vi "Text file pattern.vi"(8 "error in":errorcluster, 11 "T in":dbl) -> (0 "error out":errorcluster, 1 "selected path":path, 2 "refnum out":refnum<file>, 3 "T out":dbl)   [LabVIEW 2013]
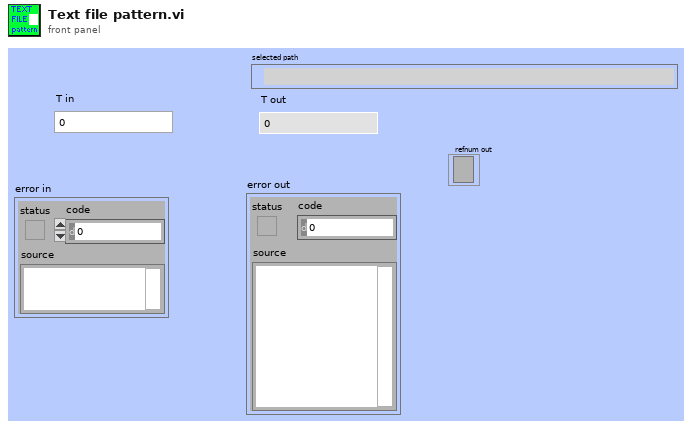
[diagram p1: front panel]
types:
  T1 = enum16{"open", "replace", "create", "open or create", "replace or create", "replace or create with confirmation"}
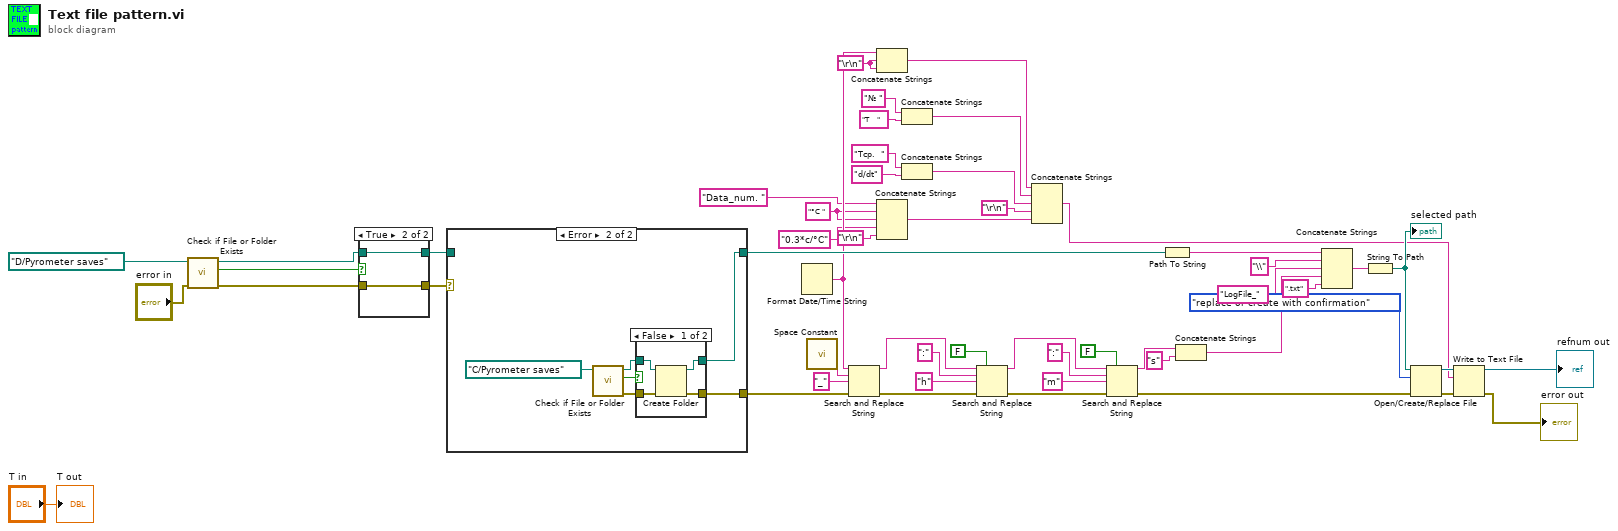
[diagram p0: block diagram]
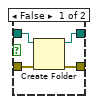
[diagram p4: hidden frame]
diagram:
  w3 = "°C " ("string")
  w8 = "\r\n"
  n1 = call <vilib>:"Check if File or Folder Exists.vi"("error in (no error)"="error in", "path"=path "D:/Pyrometer saves" ("path (use dialog)")) -> ("error out"=w31:errorcluster, "file or folder exists?"=w26:bool, "dup path"=w32:path)  [unwired: 7 out]
  n2 = case shown="True" w26 {
    tunnel: [w57 w59] -> w24
    tunnel: w32 -> [w56 w59]
    tunnel: w31 -> [w55 w58]
    tunnel: [w54 w58] -> w25
    frame False {
      n3 = Create Folder(path (use dialog)=w56, error in=w55) -> (created path=w57:path, error out=w54:errorcluster)  [unwired: 2 out]
    }
    frame True {
    }
  }
  n4 = case shown="Error" w25 {
    tunnel: w24 -> [w60 _]
    tunnel: [w60 w62] -> w23
    tunnel: [_ w61] -> w22
    frame No Error {
    }
    frame Error {
      n5 = call <vilib>:"Check if File or Folder Exists.vi"("path"=path "C:/Pyrometer saves" ("path (use dialog)")) -> ("error out"=w64:errorcluster, "file or folder exists?"=w63:bool, "dup path"=w65:path)  [unwired: 1 in, 7 out]
      n6 = case shown="False" w63 {
        tunnel: [w70 w72] -> w62
        tunnel: w65 -> [w69 w72]
        tunnel: w64 -> [w68 w71]
        tunnel: [w67 w71] -> w61
        frame False {
          n7 = Create Folder(path (use dialog)=w69, error in=w68) -> (created path=w70:path, error out=w67:errorcluster)  [unwired: 2 out]
        }
        frame True {
        }
      }
    }
  }
  n8 = Format Date/Time String() -> (date/time string=w7:string)  [unwired: 3 out]
  n9 = call <vilib>:"Space Constant.vi"() -> ("String"=w46:string)
  n10 = Search and Replace String(input string=w7, search string=w46, replace string="_" ("replace string (\"\")"), error in=w22) -> (result string=w44:string, error out=w30:errorcluster)  [unwired: 6 out]
  n11 = Concatenate Strings(w7, w8, w8) -> (w10:string)
  n12 = Concatenate Strings("Data_num. " ("string"), w3, w3, "0.3*c/°C" ("string"), "\r\n") -> (w5:string)
  n13 = Concatenate Strings("№ " ("string"), "T    " ("string")) -> (w12:string)
  n14 = Concatenate Strings("Tср.  " ("string"), "d/dt" ("string")) -> (w11:string)
  n15 = Search and Replace String(replace all?=FALSE ("replace all? (F)"), input string=w44, search string=":", replace string="h" ("replace string (\"\")"), error in=w30) -> (result string=w37:string, error out=w29:errorcluster)  [unwired: 5 out]
  n16 = Concatenate Strings(w10, w12, w11, "\r\n", w5) -> (w9:string)
  n17 = Search and Replace String(replace all?=FALSE ("replace all? (F)"), input string=w37, search string=":", replace string="m" ("replace string (\"\")"), error in=w29) -> (result string=w21:string, error out=w27:errorcluster)  [unwired: 5 out]
  n18 = Path To String(path=w23) -> (string=w35:string)
  n19 = Concatenate Strings(w21, "s" ("string")) -> (w18:string)
  n20 = Concatenate Strings(w35, "\\" ("string"), "LogFile_" ("string"), w18, ".txt" ("default name")) -> (w47:string)
  n21 = String To Path(string=w47) -> (path=w36:path)
  "selected path" <- w36
  n22 = Open/Create/Replace File(file path (use dialog)=w36, error in=w27, operation (0:open)=T1."replace or create with confirmation") -> (refnum out=w52:refnum<file>, error out=w50:errorcluster)  [unwired: 4 out]
  n23 = Write to Text File(file (use dialog)=w52, text=w9, error in=w50) -> (refnum out=→"refnum out":refnum<file>, error out=→"error out":errorcluster)  [unwired: 2 out]
  "T out" <- "T in"
